vi "Apply System Image.vi"(8 "error in":errorcluster caption="error in (no error)", 11 "Target information":T2={"Hostname"="", "Serial number"="", "Product name"="", "Product code"=0, "System status"="", "Credential type"=enum."None/Unlocked", "User added?"=FALSE, "Primary NIC"={"MAC address"="", "IP Address Request Mode"=2, "IP address"="", "Subnet mask"="", "Gateway"="", "DNS server"=""}} {"Primary NIC"."IP Address Request Mode" items=["Static"=1, "DHCP/Link-Local"=2, "Link-Local Only"=4, "DHCP Only"=8]}) -> (0 "error out":errorcluster, 3 "Real-Time:System Status":string)   [LabVIEW 2020]
doc: "Applies the most updated system image found in the local machine."
uses:
  subVIs/Targets/TypeDefs/rad_Target Network Settings.ctl
  <vilib>/nisyscfg/Network Settings Format.ctl
  <vilib>/nisyscfg/Format With Base System Image.vi
  <vilib>/nisyscfg/Close (System).vi
  <vilib>/nisyscfg/nisyscfg.lvlib
  <resource>/objmgr/nisysapi.rc
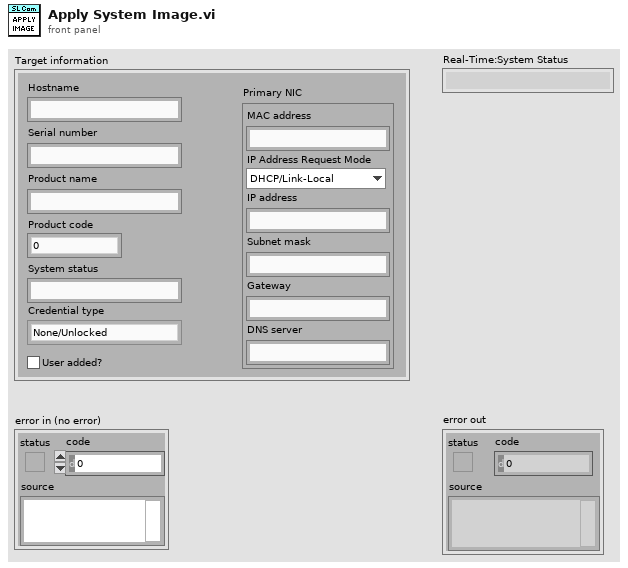
[diagram p1: front panel]
types:
  T1 = typedef "rad_Target Network Settings.ctl" = cluster{"MAC address":string, "IP Address Request Mode":i32, "IP address":string, "Subnet mask":string, "Gateway":string, "DNS server":string}
  T2 = cluster{"Hostname":string, "Serial number":string, "Product name":string, "Product code":i32, "System status":string, "Credential type":enum16{"None/Unlocked", "FTP Password", "NIAuth Credentials"}, "User added?":bool, "Primary NIC":T1}
  T3 = typedef "nisyscfg.lvlib/Network Settings Format.ctl" = u32
  T4 = typedef "nisyscfg.lvlib/Software 1.2.ctl" = cluster{"title":string, "description":string, "ID":string, "version":string, "component type":T5}
  T5 = typedef "nisyscfg.lvlib/Component Type.ctl" = u32
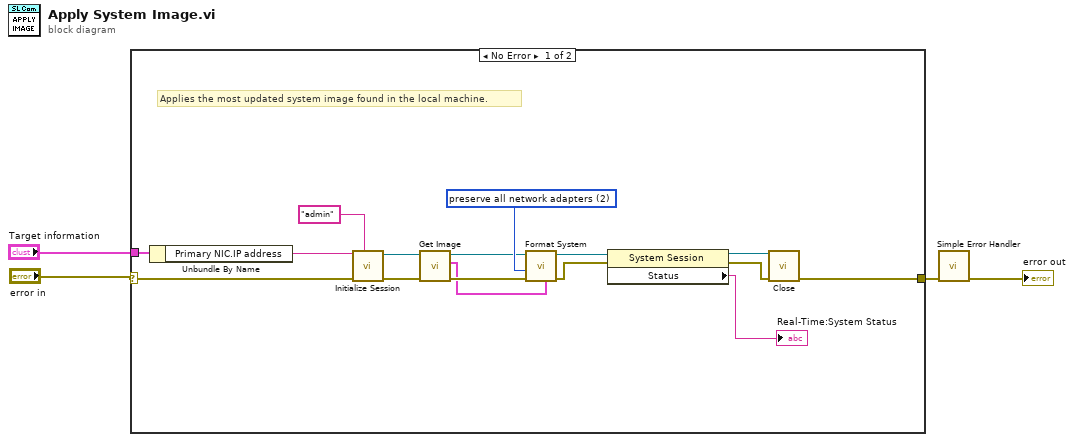
[diagram p0: block diagram]
diagram:
  n1 = case shown="No Error" "error in" {
    selector: "error in" -> [w16 w21]
    tunnel: [w20 w21] -> w2
    tunnel: "Target information" -> [w18 _]
    frame No Error {
      w15 = T3 2 items=["reset all network adapters", "preserve primary, reset others", "preserve all network adapters"] ("Network Settings (reset all adapters)")
      # "Applies the most updated system image found in the local machine."
      n2 = Unbundle By Name(w18) -> ("Primary NIC.IP address"=w17:string)
      n3 = call <vilib>:"Initialize Session.vi"("User Name"="admin", "error in (no error)"=w16, "Target (localhost)"=w17) -> ("error out"=w13:errorcluster, "Session out"=w14:refnum<k21>)  [unwired: 7 in]
      n4 = call "Get Image.vi"("error in"=w13, "Refnum in"=w14) -> ("error out"=w11:errorcluster, "element"=w10:T4, "Refnum out"=w12:refnum<k21>)  [unwired: 7 in]
      n5 = call-poly <vilib>:"Format System.vi"("Base System Image"=w10, "error in (no error)"=w11, "Network Settings (reset all adapters)"=w15, "Session in"=w12) -> ("error out"=w8:errorcluster, "Session out"=w9:refnum<k21>)  [unwired: 6 in]
      n6 = property class="System Session"(reference=w9, error in=w8) -> (reference out=w7:refnum<k21>, error out=w6:errorcluster, "Status"=→"Real-Time:System Status":string)
      n7 = call-poly <vilib>:"Close.vi"("error in (no error)"=w6, "Session in"=w7) -> ("error out"=w20:errorcluster)  [unwired: 9 in]
    }
    frame Error {
    }
  }
  n8 = call <vilib>:"Simple Error Handler.vi"("error in (no error)"=w2) -> ("error out"=→"error out":errorcluster)  [unwired: 4 in, 4 out]
